vi "Write HAL Config Data.vi"(8 "error in (no error)":errorcluster, 10 "HAL Config Data":T1, 11 "DriverMasterSync in":refnum<class "DriverMasterSync.lvclass">) -> (0 "error out":errorcluster, 3 "DriverMasterSync out":refnum<class "DriverMasterSync.lvclass">)   [LabVIEW 2014, in "DriverMasterSync.lvlib" / "DriverMasterSync.lvclass"]
uses:
  DriverMasterSync.lvclass
  TypeDefs/HAL Config Data.ctl
  DriverMasterSync.lvclass/DriverMasterSync.ctl
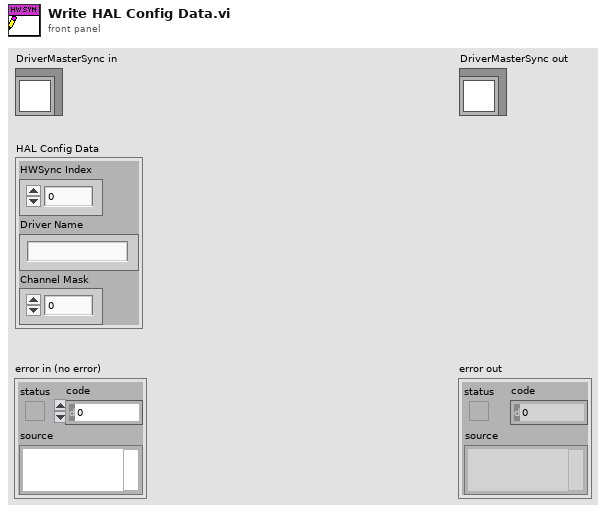
[diagram p1: front panel]
types:
  T1 = typedef "HAL Config Data.ctl" = cluster{"HWSync Index":u32, "Driver Name":string, "Channel Mask":u64}
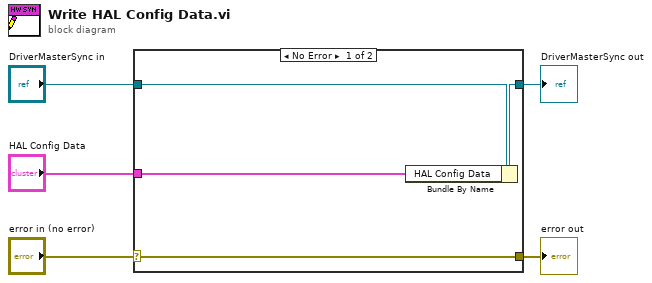
[diagram p0: block diagram]
diagram:
  n1 = case shown="No Error" "error in (no error)" {
    selector: "error in (no error)" -> [w9 w10]
    tunnel: [w9 w10] -> w4
    tunnel: [w7 w11] -> w2
    tunnel: "DriverMasterSync in" -> [w8 w11]
    tunnel: "HAL Config Data" -> [w6 _]
    frame No Error {
      n2 = Bundle By Name(cluster=w8, "HAL Config Data"=w6) -> (w7:refnum<class "DriverMasterSync.lvclass">)
    }
    frame Error {
    }
  }
  "error out" <- w4
  "DriverMasterSync out" <- w2
